vi "test_psmc_2.vi"() -> ()   [LabVIEW 2014]
uses:
  <vilib>/ptbypt/NI_PtbyPt.lvlib
panel:
  in  "Kv":dbl=5.0
  in  "Kp":dbl=0.5
  in  "pd":dbl
  out "reference vs actual":T1(graph)={"M1 desired speed"=-2.643844573044476e-06, "M1 position"=0.0002596427270612935}
  in  "stop":bool
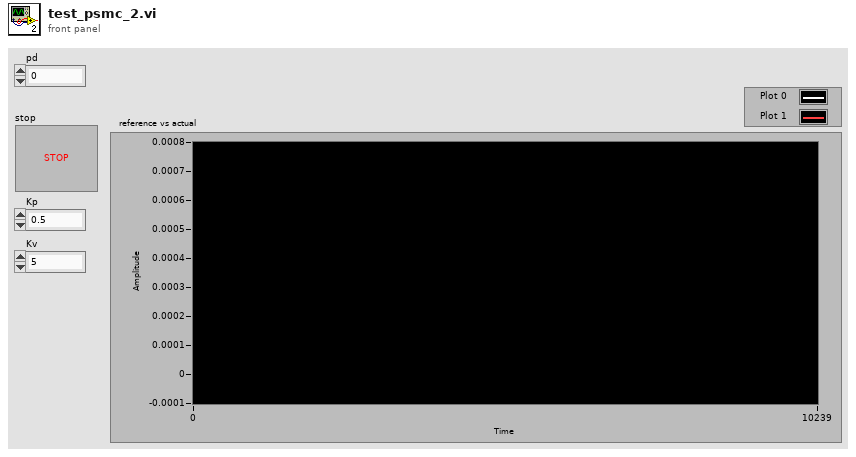
[diagram p1: front panel]
types:
  T1 = cluster{"M1 desired speed":dbl, "M1 position":dbl}
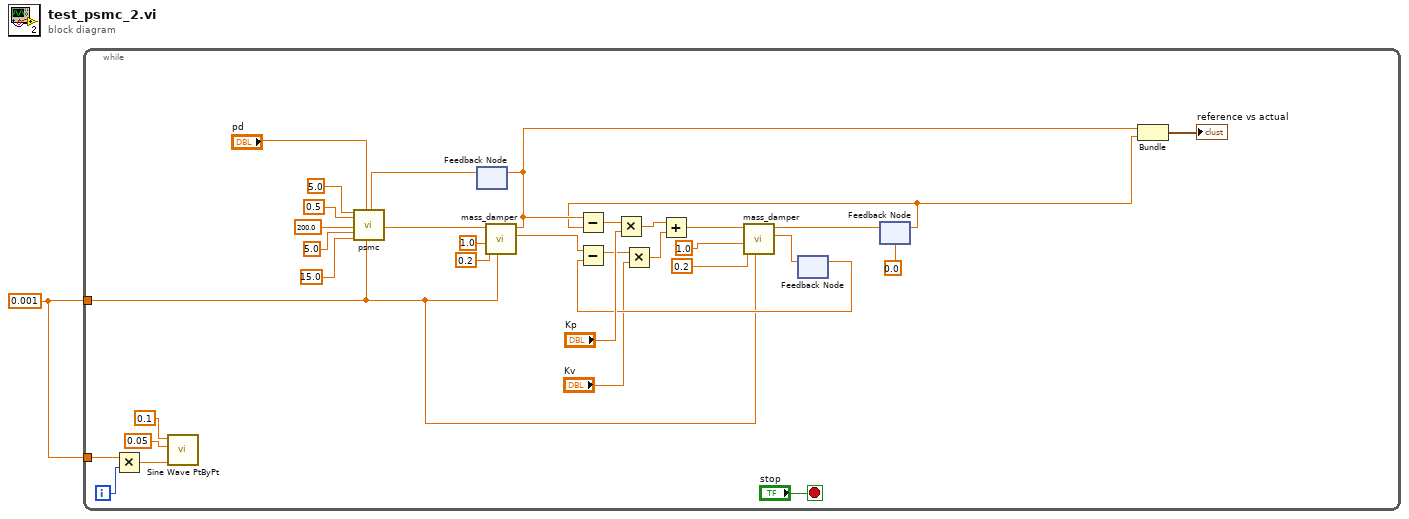
[diagram p0: block diagram]
diagram:
  w1 = 0.001 ("T")
  n1 = while {
    tunnel: w1 -> [w30]
    tunnel: w1 -> [w2]
    i -> [w31]
    stop <- "stop" stop-if-true
    n2 = Multiply(x=w30, y=w31) -> (x*y=w34:dbl)
    n3 = call <vilib>:"Sine Wave PtByPt.vi"("time"=w34, "frequency"=0.05, "amplitude"=0.1) -> ()  [unwired: 1 in, 1 out]
    n4 = feedback #1() -> (w6:dbl)  [unwired: 1 in]
    n5 = call "psmc.vi"("F"=5.0, "H"=0.5, "K"=200.0, "L"=5.0, "B"=15.0, "pd"="pd", "T"=w2, "p"=w6) -> ("f"=w22:dbl)  [unwired: 11 in]
    n6 = call "mass_damper.vi"("dt"=w2, "B"=0.2, "Mass"=1.0, "f(t)"=w22) -> ("x_dot(t)"=w16:dbl, "x(t)"=w4:dbl)  [unwired: 5 in, 1 out]
    n7 = feedback-in #1(w4) -> ()
    n8 = feedback #2() -> (w14:dbl)  [unwired: 1 in]
    n9 = Subtract(x=w16, y=w14) -> (x-y=w13:dbl)
    n10 = Multiply(x=w13, y="Kv") -> (x*y=w10:dbl)
    n11 = feedback #3(0.0 ("integral x(t)")) -> (w3:dbl)
    n12 = Subtract(x=w4, y=w3) -> (x-y=w17:dbl)
    n13 = Multiply(x=w17, y="Kp") -> (x*y=w11:dbl)
    n14 = Add(x=w11, y=w10) -> (x+y=w9:dbl)
    n15 = call "mass_damper.vi"("dt"=w2, "B"=0.2, "Mass"=1.0, "f(t)"=w9) -> ("x_dot(t)"=w15:dbl, "x(t)"=w19:dbl)  [unwired: 5 in, 1 out]
    n16 = feedback-in #2(w15) -> ()
    n17 = feedback-in #3(w19) -> ()
    n18 = Bundle("x(t)"=w4, "integral x(t)"=w3) -> (→"reference vs actual":cluster{"x(t)":dbl, "integral x(t)":dbl})  [unwired: 1 in]
  }
